vi "shooterPID.vi"(8 "pidGains":T3={"proportional gain (Kc)"=1.0, "integral time (Ti, min)"=0.01, "derivative time (Td, min)"=0.0} {"derivative time (Td, min)" format="%.3f"; "integral time (Ti, min)" format="%.3f"; "proportional gain (Kc)" format="%.3f"}, 9 "rpmTarget":dbl, 10 "CounterDevRef":T1) -> (3 "output":dbl format="%.2f")   [LabVIEW 2012]
uses:
  <vilib>/Rock Robotics/WPI/Counter/WPI_CounterDevRef.ctl
  <vilib>/Rock Robotics/SystemInterfaces/Counter/FPGA_CounterCtrSystemIndex.ctl
  <vilib>/Rock Robotics/WPI/DriverStation/DriverStationLCD/WPI_DriverStationLCDLCDLine.ctl
  <vilib>/addons/control/pid/pid.llb/PID (DBL).vi
  <vilib>/addons/control/pid/NI_PID_pid.lvlib
panel:
  out "withinRangeMotor1":bool
  in  "rpmRangeMotor1":dbl
  out "rpmCurrentMotor1":dbl
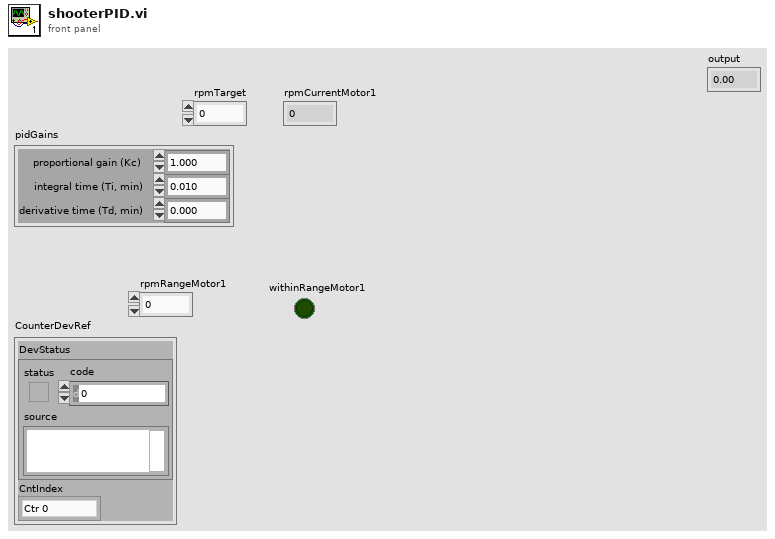
[diagram p1: front panel]
types:
  T1 = typedef "WPI_CounterDevRef.ctl" = cluster{"DevStatus":errorcluster, "CntIndex":T2}
  T2 = typedef "FPGA_CounterCtrSystemIndex.ctl" = enum8{"Ctr 0", "Ctr 1", "Ctr 2", "Ctr 3", "Ctr 4", "Ctr 5", "Ctr 6", "Ctr 7", "Invalid"}
  T3 = cluster{"proportional gain (Kc)":dbl, "integral time (Ti, min)":dbl, "derivative time (Td, min)":dbl}
  T4 = typedef "WPI_DriverStationLCDLCDLine.ctl" = enum16{"Main - Line 1", "User - Line 2", "User - Line 3", "User - Line 4", "User - Line 5", "User - Line 6"}
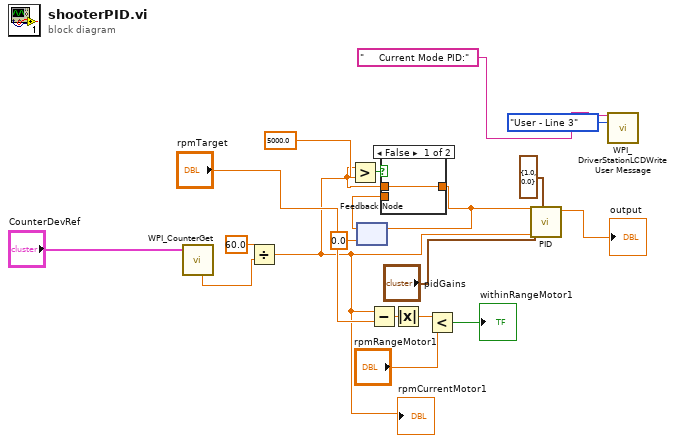
[diagram p0: block diagram]
diagram:
  n1 = call <vilib>:"WPI_CounterGet.vi"("CounterDevRef in"="CounterDevRef") -> ("Period (sec)"=w18:dbl)  [unwired: 5 in, 5 out]
  n2 = Divide(x=60.0, y=w18) -> (x/y=w3:dbl)
  "rpmCurrentMotor1" <- w3
  n3 = Greater?(x=w3, y=5000.0) -> (0:w8:bool)
  n4 = feedback #1(0.0 ("rpmTarget")) -> (w6:dbl)
  n5 = Subtract(x=w3, y="rpmTarget") -> (x-y=w15:dbl)
  n6 = case shown="False" w8 {
    tunnel: w3 -> [w20 _]
    tunnel: [w20 w21] -> w5
    tunnel: w6 -> [_ w21]
    frame False {
    }
    frame True {
    }
  }
  n7 = feedback-in #1(w5) -> ()
  n8 = Absolute Value(x=w15) -> (abs(x)=w14:dbl)
  n9 = Less?(x=w14, y="rpmRangeMotor1") -> (x < y?=→"withinRangeMotor1":bool)
  n10 = call-poly <vilib>:"PID.vi"("output range"=cluster{"output high":dbl, "output low":dbl} {"output high"=1.0, "output low"=0.0}, "PID gains"="pidGains", "process variable"=w3, "setpoint"=w5) -> ("output"=→"output":dbl)  [unwired: 6 in, 1 out]
  n11 = call <vilib>:"WPI_DriverStationLCDWrite User Message.vi"("line text"="     Current Mode PID:" ("string"), "line"=WPI_DriverStationLCDLCDLine."User - Line 3") -> ()  [unwired: 13 in, 1 out]
